vi "Compute Destination Endpoints.vi"(8 "error in (no error)":errorcluster, 9 "Endpoints":string[](array[string]), 10 "Source Endpoint":string, 11 "Refnum in":T1) -> (0 "error out":errorcluster, 2 "Possible Destination Endpoints":string[](array[string]), 3 "Refnum out":T1)   [LabVIEW 2017, in "SLSC Switch Scripting.lvlib"]
uses:
  SLSC Switch Scripting.lvlib
  <vilib>/userdefined/High Color/SLSC_Switch/nislscslSession.ctl
  <vilib>/SLSC_Switch/Path Capability.ctl
  <vilib>/SLSC_Switch/SLSC Switch.lvlib
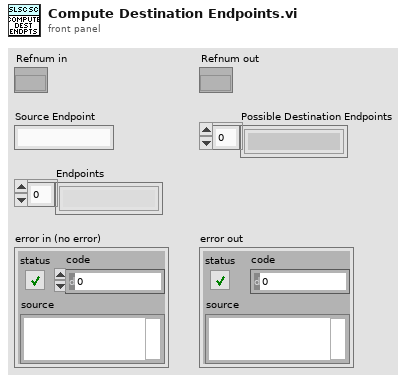
[diagram p1: front panel]
types:
  T1 = typedef "nislscslSession.ctl" = refnum<k20>
  T2 = typedef "SLSC Switch.lvlib/Path Capability.ctl" = i32
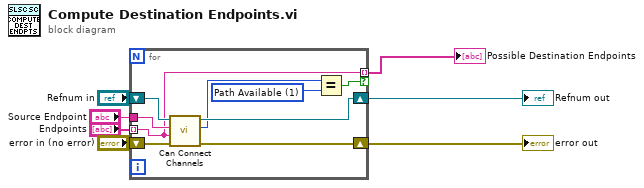
[diagram p0: block diagram]
diagram:
  n1 = for {
    tunnel: "Endpoints" -> [w9] mode=indexing
    shift-right: [w15] -> w3
    shift-left: "error in (no error)" -> [w16]
    shift-right: [w13] -> w5
    shift-left: "Refnum in" -> [w14]
    tunnel: "Source Endpoint" -> [w12]
    tunnel: [w9] -> w7 mode=indexing if=w8
    w10 = T2 1 items=["Path Available"=1, "Path Exists"=2, "Path Unsupported"=3, "Resource in Use"=4, "Source Conflict"=5, "Channel Not Available"=6] ("y")
    n2 = call <vilib>:"Can Connect Channels.vi"("error in (no error)"=w16, "channel 2"=w9, "channel 1"=w12, "session in"=w14) -> ("error out"=w15:errorcluster, "path capability"=w11:T2, "session out"=w13:T1)  [unwired: 5 in]
    n3 = Equal?(x=w11, y=w10) -> (x = y?=w8:bool)
  }
  "Possible Destination Endpoints" <- w7
  "Refnum out" <- w5
  "error out" <- w3
